vi "Power Values.vi"   [LabVIEW 2014, in "NI_EP_Power Quality.lvlib"]
doc: "Calculates the power values from the voltage and current spectra of different line configurations. You must manually select the polymorphic instance you want to use."
uses:
  <vilib>/addons/Electrical Power/PQ/NI_EP_Power Quality.lvlib
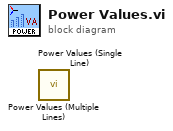
[diagram p0: block diagram]
diagram:
  n1 = call <vilib>:"Power Values (Multiple Lines).vi"() -> ()  [unwired: 12 in, 4 out]
  n2 = call <vilib>:"Power Values (Single Line).vi"() -> ()  [unwired: 12 in, 4 out]
